vi "ForceTimeAlign.vi"(0 "DUTDataArray":T8[](array[typedef]) {"TimeStamp" format="%^<%.3X\n%x>T"; "Time" format="%.6f"}, 1 "NIAnalysisArray":T1[](array[typedef]) {"Time" format="%.6f"; "TimeStamp" format="%^<%.3X\n%x>T"}, 5 "NIDataArray":T6 {"TimeStamp" format="%^<%.3X\n%x>T"; "Time" format="%.6f"}, 7 "PMUDataArray":T3[](array[typedef]) {"FREQUENCY" format="%#_6f"; "TimeStamp" format="%^<%.3X\n%x>T"}, 9 "DataAnalysisArray":T5[](array[typedef]) {"TimeStamp" format="%^<%.3X\n%x>T"}, 11 "ModelDataArray":T3[](array[typedef]) {"FREQUENCY" format="%#_6f"; "TimeStamp" format="%^<%.3X\n%x>T"}, 12 "error in (no error)":errorcluster) -> (3 "NIAnalysisArray 2":T1[](array[typedef]) {"Time" format="%.6f"; "TimeStamp" format="%^<%.3X\n%x>T"}, 4 "DUTDataArray":T8[](array[typedef]) {"TimeStamp" format="%^<%.3X\n%x>T"; "Time" format="%.6f"}, 6 "NIDataArray":T6 {"TimeStamp" format="%^<%.3X\n%x>T"; "Time" format="%.6f"}, 8 "PMUDataArray":T3[](array[typedef]) {"FREQUENCY" format="%#_6f"; "TimeStamp" format="%^<%.3X\n%x>T"}, 10 "DataAnalysisArray":T5[](array[typedef]) {"TimeStamp" format="%^<%.3X\n%x>T"}, 14 "error out":errorcluster, 15 "ModelDataArray":T3[](array[typedef]) {"FREQUENCY" format="%#_6f"; "TimeStamp" format="%^<%.3X\n%x>T"})   [LabVIEW 2014]
uses:
  typedefs/DUTData.ctl
  typedefs/PhasorRectangular.ctl
  typedefs/PmuRawDataCluster.ctl
  typedefs/NIDataArray.ctl
  typedefs/NIData.ctl
  typedefs/CalcAnalysis.ctl
  typedefs/CalcPhasorError.ctl
  typedefs/NICalcAnalysis.ctl
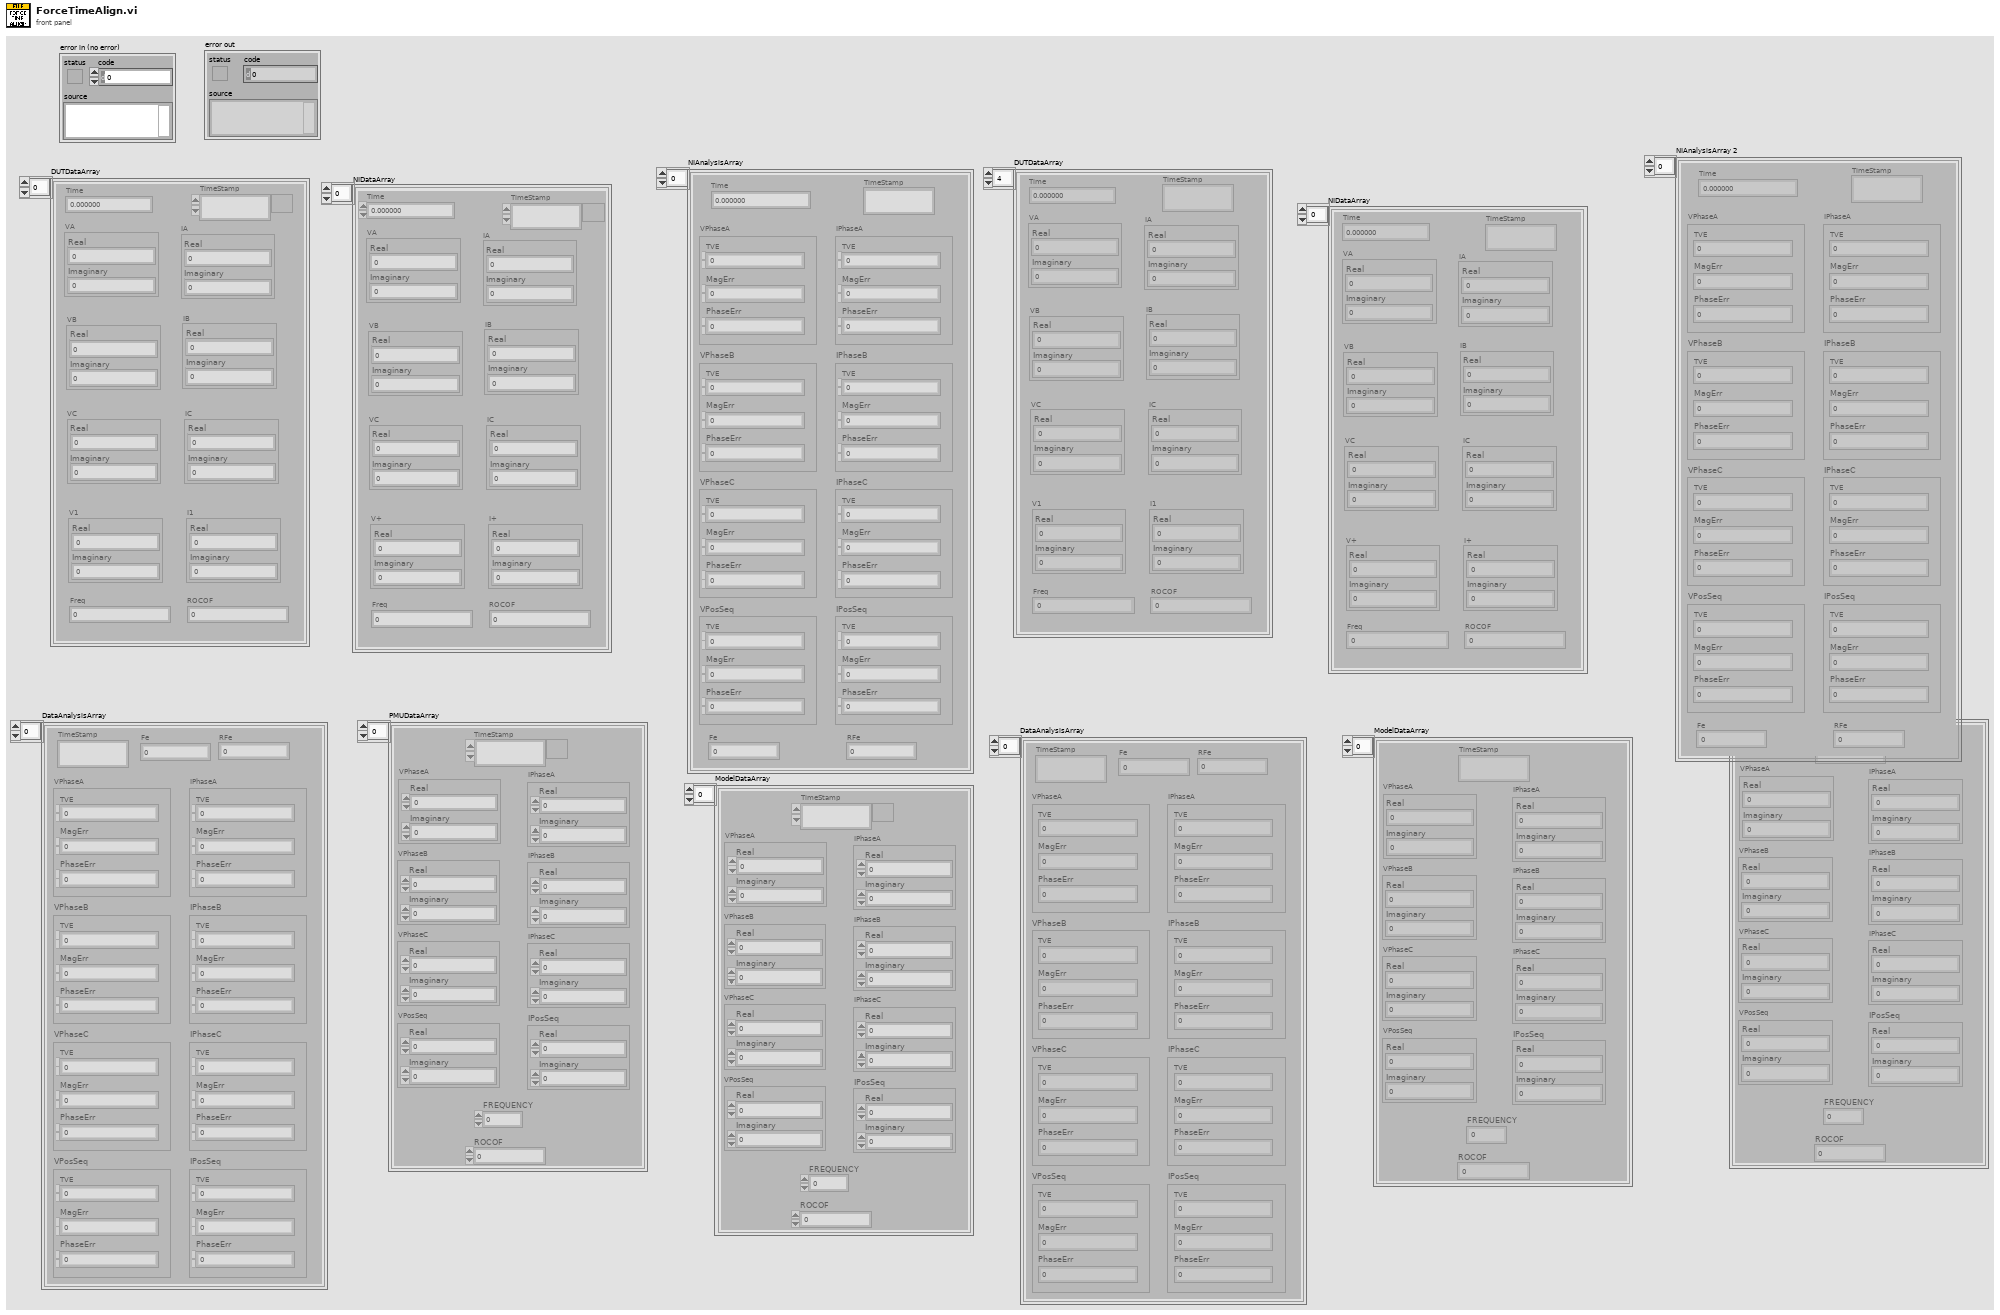
[diagram p1: front panel]
types:
  T1 = typedef "NICalcAnalysis.ctl" = cluster{"Time":dbl, "VPhaseA":T2, "VPhaseB":T2, "VPhaseC":T2, "VPosSeq":T2, "IPhaseA":T2, "IPhaseB":T2, "IPhaseC":T2, "IPosSeq":T2, "Fe":dbl, "RFe":dbl, "TimeStamp":timestamp}
  T2 = typedef "CalcPhasorError.ctl" = cluster{"TVE":dbl, "MagErr":dbl, "PhaseErr":dbl}
  T3 = typedef "PmuRawDataCluster.ctl" = cluster{"TimeStamp":timestamp, "VPhaseA":T4, "VPhaseB":T4, "VPhaseC":T4, "VPosSeq":T4, "IPhaseA":T4, "IPhaseB":T4, "IPhaseC":T4, "IPosSeq":T4, "FREQUENCY":dbl, "ROCOF":sgl}
  T4 = typedef "PhasorRectangular.ctl" = cluster{"Real":dbl, "Imaginary":dbl}
  T5 = typedef "CalcAnalysis.ctl" = cluster{"TimeStamp":timestamp, "VPhaseA":T2, "VPhaseB":T2, "VPhaseC":T2, "VPosSeq":T2, "IPhaseA":T2, "IPhaseB":T2, "IPhaseC":T2, "IPosSeq":T2, "Fe":dbl, "RFe":dbl}
  T6 = typedef "NIDataArray.ctl" = T7[]
  T7 = typedef "NIData.ctl" = cluster{"Time":dbl, "VA":T4, "VB":T4, "VC":T4, "V+":T4, "IA":T4, "IB":T4, "IC":T4, "I+":T4, "Freq":dbl, "ROCOF":dbl, "TimeStamp":timestamp}
  T8 = typedef "DUTData.ctl" = cluster{"Time":dbl, "VA":T4, "VB":T4, "VC":T4, "V1":T4, "IA":T4, "IB":T4, "IC":T4, "I1":T4, "Freq":dbl, "ROCOF":dbl, "TimeStamp":timestamp}
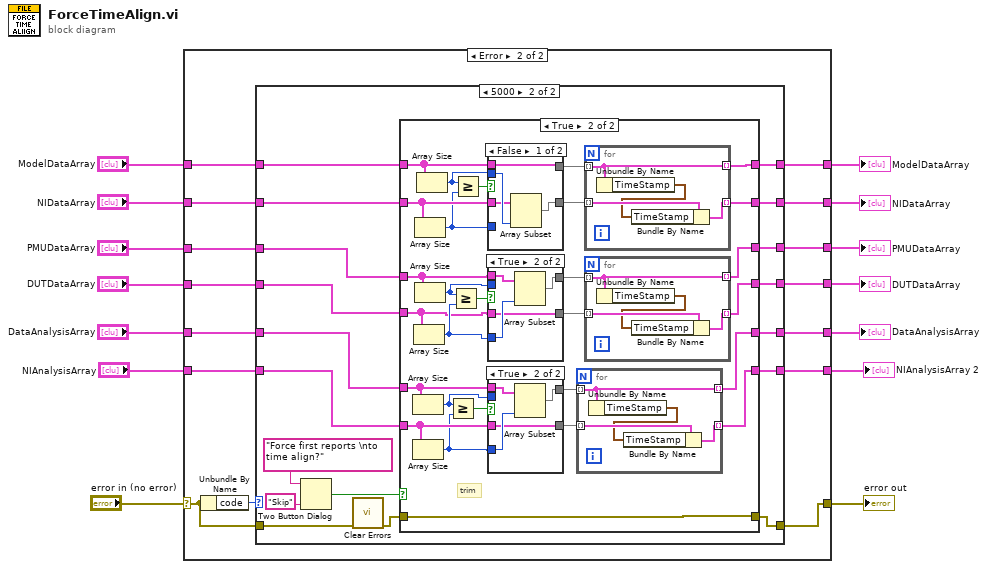
[diagram p0: block diagram]
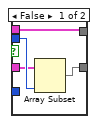
[diagram p5: hidden frame]
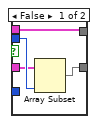
[diagram p6: hidden frame]
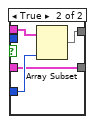
[diagram p7: hidden frame]
diagram:
  n1 = case shown="Error" "error in (no error)" {
    selector: "error in (no error)" -> [w21 w35]
    tunnel: [w21 w34] -> w13
    tunnel: "DUTDataArray" -> [w20 w33]
    tunnel: "NIDataArray" -> [w19 w32]
    tunnel: "PMUDataArray" -> [w18 w31]
    tunnel: "DataAnalysisArray" -> [w17 w30]
    tunnel: "ModelDataArray" -> [w16 w29]
    tunnel: [w20 w28] -> w7
    tunnel: [w19 w27] -> w6
    tunnel: [w18 w26] -> w5
    tunnel: [w17 w25] -> w4
    tunnel: [w16 w24] -> w3
    tunnel: [w15 w23] -> w2
    tunnel: "NIAnalysisArray" -> [w15 w22]
    frame No Error {
    }
    frame Error {
      n2 = Unbundle By Name(w35) -> ("code"=w36:i32)
      n3 = case shown="5000" w36 {
        tunnel: w35 -> [w43 w45]
        tunnel: [w43 w59] -> w34
        tunnel: w33 -> [w42 w58]
        tunnel: w32 -> [w41 w57]
        tunnel: w31 -> [w40 w56]
        tunnel: w30 -> [w39 w55]
        tunnel: w29 -> [w38 w54]
        tunnel: [w42 w53] -> w28
        tunnel: [w41 w52] -> w27
        tunnel: [w40 w51] -> w26
        tunnel: [w39 w50] -> w25
        tunnel: [w38 w49] -> w24
        tunnel: [w37 w48] -> w23
        tunnel: w22 -> [w37 w47]
        frame 0, Default {
        }
        frame 5000 {
          n4 = Two Button Dialog(message="Force first reports \nto time align?", 1:"Skip" ("F button name (\"Cancel\")")) -> (T button?=w60:bool)  [unwired: 1 in]
          n5 = call <vilib>:"Clear Errors.vi"("error in (no error)"=w45) -> ("error out"=w44:errorcluster)  [unwired: 5 in, 1 out]
          n6 = case shown="True" w60 {
            tunnel: w44 -> [w68 w69]
            tunnel: [w68 w69] -> w59
            tunnel: w58 -> [w67 w87]
            tunnel: w57 -> [w66 w94]
            tunnel: w56 -> [w65 w91]
            tunnel: w55 -> [w64 w86]
            tunnel: w54 -> [w63 w95]
            tunnel: [w67 w74] -> w53
            tunnel: [w66 w78] -> w52
            tunnel: [w65 w75] -> w51
            tunnel: [w64 w71] -> w50
            tunnel: [w63 w79] -> w49
            tunnel: [w62 w70] -> w48
            tunnel: w47 -> [w62 w85]
            frame False {
            }
            frame True {
              # "trim"
              n7 = Array Size(array=w86) -> (size(s)=w83:i32)
              n8 = Array Size(array=w85) -> (size(s)=w82:i32)
              n9 = Array Size(array=w87) -> (size(s)=w88:i32)
              n10 = Array Size(array=w94) -> (size(s)=w93:i32)
              n11 = Array Size(array=w91) -> (size(s)=w89:i32)
              n12 = Array Size(array=w95) -> (size(s)=w92:i32)
              n13 = Greater Or Equal?(x=w83, y=w82) -> (x >= y?=w84:bool)
              n14 = Greater Or Equal?(x=w89, y=w88) -> (x >= y?=w90:bool)
              n15 = Greater Or Equal?(x=w92, y=w93) -> (x >= y?=w96:bool)
              n16 = case shown="False" w96 {
                tunnel: w95 -> [w126 w131]
                tunnel: w94 -> [w127 w130]
                tunnel: w93 -> [_ w132]
                tunnel: w92 -> [w128 _]
                tunnel: [w125 w130] -> w80
                tunnel: [w126 w129] -> w81
                frame False {
                  n17 = Array Subset(array=w127, length=w128) -> (w125:T6)  [unwired: 1 in]
                }
                frame True {
                  n18 = Array Subset(array=w131, length=w132) -> (w129:T3[])  [unwired: 1 in]
                }
              }
              n19 = case shown="True" w90 {
                tunnel: w91 -> [w118 w123]
                tunnel: w87 -> [w119 w122]
                tunnel: w88 -> [_ w124]
                tunnel: w89 -> [w120 _]
                tunnel: [w117 w122] -> w73
                tunnel: [w118 w121] -> w77
                frame False {
                  n20 = Array Subset(array=w119, length=w120) -> (w117:T8[])  [unwired: 1 in]
                }
                frame True {
                  n21 = Array Subset(array=w123, length=w124) -> (w121:T3[])  [unwired: 1 in]
                }
              }
              n22 = case shown="True" w84 {
                tunnel: w86 -> [w110 w115]
                tunnel: w85 -> [w111 w114]
                tunnel: w82 -> [_ w116]
                tunnel: w83 -> [w112 _]
                tunnel: [w109 w114] -> w72
                tunnel: [w110 w113] -> w76
                frame False {
                  n23 = Array Subset(array=w111, length=w112) -> (w109:T1[])  [unwired: 1 in]
                }
                frame True {
                  n24 = Array Subset(array=w115, length=w116) -> (w113:T5[])  [unwired: 1 in]
                }
              }
              n25 = for {
                tunnel: w76 -> [w98] mode=indexing
                tunnel: w72 -> [w100] mode=indexing
                tunnel: [w98] -> w71 mode=indexing
                tunnel: [w97] -> w70 mode=indexing
                n26 = Unbundle By Name(w98) -> ("TimeStamp"=w99:timestamp)
                n27 = Bundle By Name(cluster=w100, "TimeStamp"=w99) -> (w97:T1)
              }
              n28 = for {
                tunnel: w81 -> [w106] mode=indexing
                tunnel: w80 -> [w108] mode=indexing
                tunnel: [w106] -> w79 mode=indexing
                tunnel: [w105] -> w78 mode=indexing
                n29 = Unbundle By Name(w106) -> ("TimeStamp"=w107:timestamp)
                n30 = Bundle By Name(cluster=w108, "TimeStamp"=w107) -> (w105:T7)
              }
              n31 = for {
                tunnel: w77 -> [w102] mode=indexing
                tunnel: w73 -> [w104] mode=indexing
                tunnel: [w102] -> w75 mode=indexing
                tunnel: [w101] -> w74 mode=indexing
                n32 = Unbundle By Name(w102) -> ("TimeStamp"=w103:timestamp)
                n33 = Bundle By Name(cluster=w104, "TimeStamp"=w103) -> (w101:T8)
              }
            }
          }
        }
      }
    }
  }
  "error out" <- w13
  "DUTDataArray" <- w7
  "NIDataArray" <- w6
  "PMUDataArray" <- w5
  "DataAnalysisArray" <- w4
  "ModelDataArray" <- w3
  "NIAnalysisArray 2" <- w2
